vi "Read_MNK_Temp_from_DSC.vi"(8 "Read from DSC in":errorcluster) -> (0 "Read from DSC":errorcluster, 2 "Temp":dbl)   [LabVIEW 2016]
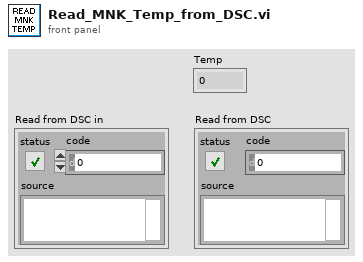
[diagram p1: front panel]
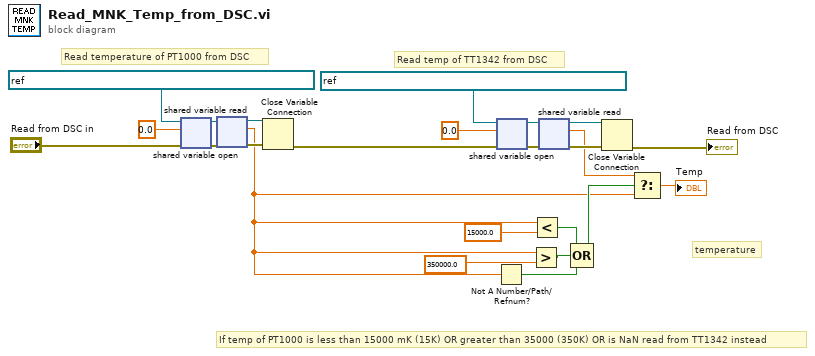
[diagram p0: block diagram]
diagram:
  # "If temp of PT1000 is less than 15000 mK (15K) OR greater than 35000 (350K) OR is NaN read from TT1342 instead"
  # "Read temp of TT1342 from DSC"
  # "Read temperature of PT1000 from DSC"
  # "temperature"
  n1 = shared-variable-open(refnum<k21> "ni.var.psp://housesoftheholy/MNK_18T/MNK_TC_T4" ("shared variable refnum in"), "Read from DSC in", 0.0) -> (w23:refnum<k21>, w22:errorcluster)  [unwired: 1 in]
  n2 = shared-variable-read(w23, w22) -> (w15:refnum<k21>, w21:errorcluster, w2:dbl)  [unwired: 1 out]
  n3 = Close Variable Connection(8:w21, 11:w15) -> (0:w9:errorcluster)
  n4 = Not A Number/Path/Refnum?(number/path/refnum=w2) -> (NaN/Path/Refnum?=w6:bool)
  n5 = shared-variable-open(refnum<k21> "ni.var.psp://housesoftheholy/MNK_18T/MNK_TC_T3" ("shared variable refnum in"), w9, 0.0) -> (w17:refnum<k21>, w18:errorcluster)  [unwired: 1 in]
  n6 = Greater?(x=w2, y=350000.0) -> (0:w3:bool)
  n7 = Less?(x=w2, y=15000.0) -> (x < y?=w7:bool)
  n8 = shared-variable-read(w17, w18) -> (w14:refnum<k21>, w19:errorcluster, w11:dbl)  [unwired: 1 out]
  n9 = Compound Arithmetic op=OR(w7, w3, w6) -> (w5:bool)
  n10 = Close Variable Connection(8:w19, 11:w14) -> (0:→"Read from DSC":errorcluster)
  n11 = Select(t=w11, s=w5, f=w2) -> (s? t:f=→"Temp":dbl)
